vi "Get Existing Values.vi"(0 "References":T2, 11 "error in (no error)":errorcluster) -> (4 "References out":T2, 6 "Replace existing":bool, 8 "DB File Path":string="/home/lvuser/sqlite.db", 10 "Table Name":string, 14 "Target Type":T1, 15 "error out":errorcluster)   [LabVIEW 2014, in "SQLite editor node.lvclass"]
uses:
  SQLite editor node.lvclass
  <vilib>/NI/DCAF/Tag Editor Core/Table API/Table Manager/object ref.ctl
  <vilib>/NI/DCAF/Tag Editor Core/Configuration Editor/Classes/Engine Parent/Engine Parent Editor Node.lvclass
  <vilib>/NI/DCAF/Tag Editor Core/Configuration Editor/Classes/Module editor node/module editor node.lvclass
  <vilib>/NI/Tag Bus Module Framework/root configuration/Target Types.ctl
  module/configuration/SQLite configuration.lvclass
  <vilib>/NI/Configuration Framework/serializable configuration/NISE_CEF_serializable configuration.lvclass
  <vilib>/NI/DCAF/Tag Editor Core/Table API/Table Manager/Table Manager.lvclass
  <vilib>/NI/Tag Bus Module Framework/root configuration/TBM configuration.lvclass
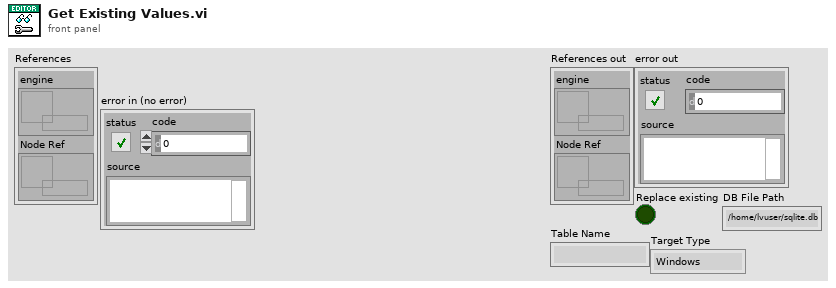
[diagram p1: front panel]
types:
  T1 = typedef "TBM configuration.lvclass/Target Types.ctl" = enum16{"Windows", "Mac", "Linux", "Linux RT ARM", "VxWorks", "Pharlap", "Other", "Linux RT x64"}
  T2 = typedef "Table Manager.lvlib/Table Manager.lvclass/object ref.ctl" = cluster{"engine":refnum<data-value>, "Node Ref":refnum<data-value>}
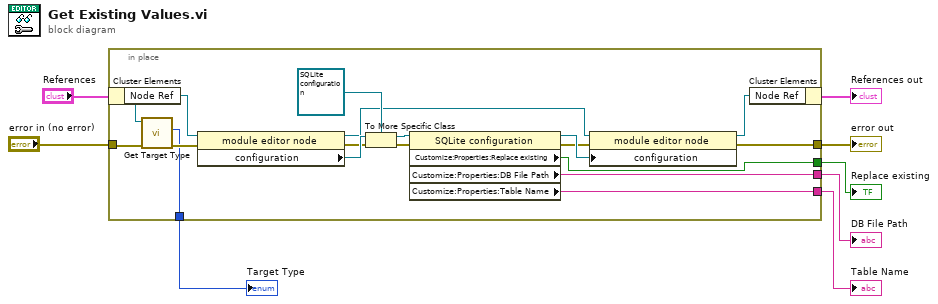
[diagram p0: block diagram]
diagram:
  n1 = in-place {
    in-place-border: "error in (no error)" -> [w12]
    in-place-border: [w16] -> w5
    in-place-border: [w15] -> w4
    in-place-border: [w14] -> w3
    in-place-border: [w13] -> w2
    in-place-border: [w10] -> w1
    n2 = in-place-cluster #1("References") -> ("Node Ref"=w9:refnum<data-value>)
    n3 = call "Get Target Type.vi"("error in (no error)"=w12, "node ref in"=w9) -> ("error out"=w11:errorcluster, "Target Type"=w10:T1)  [unwired: 7 in, 1 out]
    n4 = property class="module editor node"(reference=w9, error in=w11) -> (reference out=w19:refnum<data-value>, error out=w23:errorcluster, "configuration"=w25:refnum<class "NISE_CEF_serializable configuration.lvclass">)
    n5 = To More Specific Class(target class=refnum<class "SQLite configuration.lvclass"> refnum ("SQLite configuration"), reference=w25, error in=w23) -> (specific class reference=w22:refnum<class "SQLite configuration.lvclass">, error out=w21:errorcluster)
    n6 = property class="SQLite configuration"(reference=w22, error in=w21) -> (reference out=w20:refnum<class "SQLite configuration.lvclass">, error out=w18:errorcluster, "Customize:Properties:Replace existing"=w15:bool, "Customize:Properties:DB File Path"=w13:string, "Customize:Properties:Table Name"=w14:string)
    n7 = property class="module editor node"(reference=w19, error in=w18, "configuration"=w20) -> (reference out=w17:refnum<data-value>, error out=w16:errorcluster)
    n8 = in-place-cluster #1("Node Ref"=w17) -> (→"References out":T2)
  }
  "error out" <- w5
  "Replace existing" <- w4
  "DB File Path" <- w2
  "Table Name" <- w3
  "Target Type" <- w1
